vi "readVarillaDataInVarillaTable.vi"(8 "error in":errorcluster, 11 "dataToQueryOfRead":T1) -> (0 "error out":errorcluster, 3 "ClusterFormat":T1)   [LabVIEW 2014]
uses:
  <vilib>/addons/database/Connection.llb/DB Tools Open Connec (String).vi
  <vilib>/addons/database/Auxilliary.llb/DB Tools Format Datetime String (Time Stamp).vi
  <vilib>/addons/database/NI_Database_API.lvlib
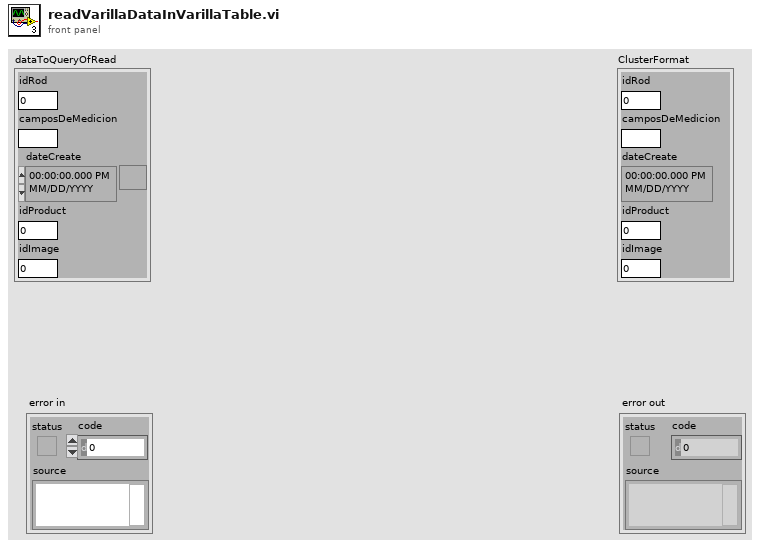
[diagram p1: front panel]
types:
  T1 = cluster{"idRod":dbl, "camposDeMedicion":string, "dateCreate":timestamp, "idProduct":dbl, "idImage":dbl}
  T2 = typedef "NI_Database_API.lvlib/Conn ObjectReference.ctl" = refnum<k1>
  T3 = typedef "NI_Database_API.lvlib/DB Tools DataTypes.ctl" = enum16{"String", "Long (I32)", "Single (SGL)", "Double (DBL)", "Date/Time", "Binary"}
  T4 = cluster{"name":string, "database data type":T3, "defined size":i32}[]
  T5 = cluster{string, "camposDeMedicion":string, "date/time string":string, string, string}
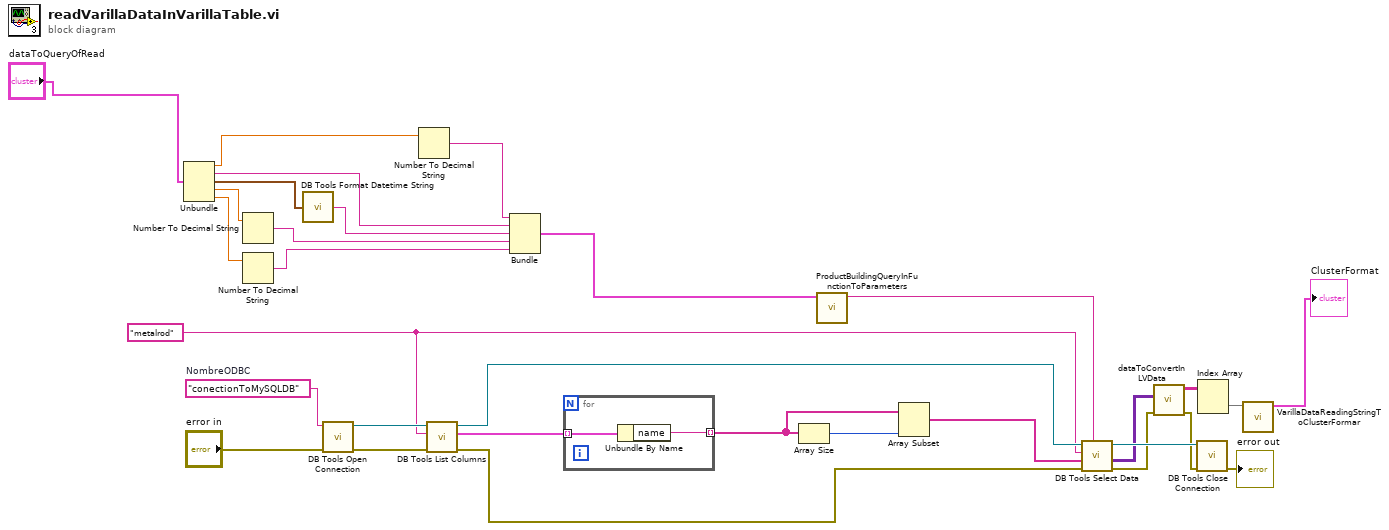
[diagram p0: block diagram]
diagram:
  w18 = "metalrod" ("tableName")
  w31 = "conectionToMySQLDB"  # NombreODBC
  n1 = Unbundle("dataToQueryOfRead") -> ("idRod"=w25:dbl, "camposDeMedicion"=w24:string, "dateCreate"=w3:timestamp, "idProduct"=w5:dbl, "idImage"=w7:dbl)
  n2 = Number To Decimal String(number=w5) -> (decimal integer string=w4:string)  [unwired: 1 in]
  n3 = Number To Decimal String(number=w7) -> (decimal integer string=w6:string)  [unwired: 1 in]
  n4 = call-poly <vilib>:"DB Tools Format Datetime String.vi"("time stamp"=w3) -> ("date/time string"=w2:string)
  n5 = call-poly <vilib>:"DB Tools Open Connection.vi"("error in (no error)"="error in", "connection information"=w31) -> ("error out"=w29:errorcluster, "connection reference"=w30:T2)  [unwired: 6 in]
  n6 = Number To Decimal String(number=w25) -> (decimal integer string=w26:string)  [unwired: 1 in]
  n7 = call <vilib>:"DB Tools List Columns.vi"("error in (no error)"=w29, "table"=w18, "connection reference"=w30) -> ("error out"=w19:errorcluster, "column information"=w27:T4, "connection reference out"=w20:T2)  [unwired: 1 in, 1 out]
  n8 = Bundle(w26, "camposDeMedicion"=w24, "date/time string"=w2, w4, w6) -> (w1:T5)  [unwired: 1 in]
  n9 = for {
    tunnel: w27 -> [w33] mode=indexing
    tunnel: [w32] -> w22 mode=indexing
    n10 = Unbundle By Name(w33) -> ("name"=w32:string)
  }
  n11 = Array Size(array=w22) -> (size(s)=w23:i32)
  n12 = call "ProductBuildingQueryInFunctionToParameters.vi"("ParameterToRead"=w1) -> ("QueryToRead"=w17:string)  [unwired: 10 in]
  n13 = Array Subset(array=w22, length=w23) -> (w21:string[])  [unwired: 1 in]
  n14 = call <vilib>:"DB Tools Select Data.vi"("condition"=w17, "error in (no error)"=w19, "columns"=w21, "table"=w18, "connection reference"=w20) -> ("error out"=w13:errorcluster, "data"=w14:variant[][], "connection reference out"=w16:T2)  [unwired: 1 in]
  n15 = call "dataToConvertInLVData.vi"("error in"=w13, "dataReadingIn"=w14) -> ("error out"=w12:errorcluster, "dataReadingOut"=w11:string[][])  [unwired: 8 in]
  n16 = call <vilib>:"DB Tools Close Connection.vi"("error in (no error)"=w12, "connection reference"=w16) -> ("error out"=→"error out":errorcluster)  [unwired: 5 in]
  n17 = Index Array(array=w11) -> (element=w10:string[])  [unwired: 2 in]
  n18 = call "VarillaDataReadingStringToClusterFormar.vi"("StringFormat"=w10) -> ("ClusterFormat"=→"ClusterFormat":T1)  [unwired: 10 in]
